vi "getLastRowAndLastColumn.vi"(8 "error in (no error)":errorcluster, 11 "MS-Excel in":refnum<class "MS-Excel.lvclass">) -> (0 "error out":errorcluster, 1 "Last Column":i32, 2 "Last Row":i32, 3 "MS-Excel out":refnum<class "MS-Excel.lvclass">)   [LabVIEW 2017, in "LabVIEW NPOI.lvlib" / "MS-Excel.lvclass"]
uses:
  MS-Excel.lvclass
  C:/Users/Neo/Desktop/Dev_Tools_BR/LabVIEW_NPOI/lib/NPOI 2.1.1/NPOI.dll
  lib/NPOI 2.1.1/NPOI.dll
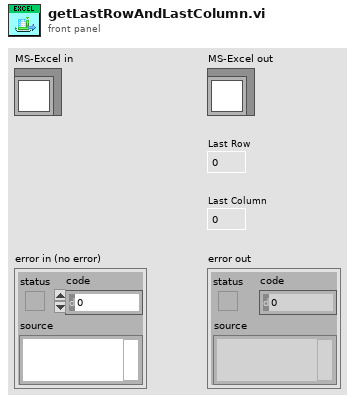
[diagram p1: front panel]
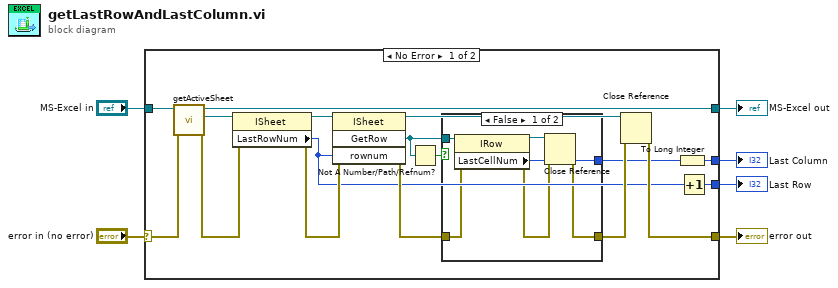
[diagram p0: block diagram]
diagram:
  n1 = case shown="No Error" "error in (no error)" {
    selector: "error in (no error)" -> [w16 w32]
    tunnel: [w14 w32] -> w5
    tunnel: [w22 w31] -> w3
    tunnel: "MS-Excel in" -> [w23 w31]
    tunnel: [w8 _] -> w2
    tunnel: [w7 _] -> w1
    frame No Error {
      n2 = call-dynamic "getActiveSheet.vi"("error in (no error)"=w16, "MS-Excel in"=w23) -> ("error out"=w19:errorcluster, "Sheet Ref"=w21:refnum<k24>, "MS-Excel out"=w22:refnum<class "MS-Excel.lvclass">)  [unwired: 6 in, 1 out]
      n3 = property class="ISheet"(reference=w21, error in=w19) -> (reference out=w20:refnum<k24>, error out=w18:errorcluster, "LastRowNum"=w13:i32)
      n4 = invoke class="ISheet" method="GetRow"(reference=w20, error in=w18, "rownum"=w13) -> (reference out=w11:refnum<k24>, error out=w17:errorcluster, "GetRow"=w9:refnum<k24>)  [unwired: 1 in, 1 out]
      n5 = Not A Number/Path/Refnum?(number/path/refnum=w9) -> (NaN/Path/Refnum?=w10:bool)
      n6 = case shown="False" w10 {
        tunnel: w9 -> [w29 _]
        tunnel: w17 -> [w28 w30]
        tunnel: [w25 w30] -> w15
        tunnel: [w24 _] -> w12
        frame False {
          n7 = property class="IRow"(reference=w29, error in=w28) -> (reference out=w26:refnum<k24>, error out=w27:errorcluster, "LastCellNum"=w24:i16)
          n8 = Close Reference(reference=w26, error in (no error)=w27) -> (error out=w25:errorcluster)
        }
        frame True {
        }
      }
      n9 = Close Reference(reference=w11, error in (no error)=w15) -> (error out=w14:errorcluster)
      n10 = To Long Integer(number=w12) -> (32bit integer=w7:i32)
      n11 = Increment(x=w13) -> (x+1=w8:i32)
    }
    frame Error {
    }
  }
  "error out" <- w5
  "MS-Excel out" <- w3
  "Last Row" <- w2
  "Last Column" <- w1
